vi "nivision_savepng.vi"(6 "Use bit depth? (false)":bool, 7 "Color Palette":cluster{"Red":u8, "Green":u8, "Blue":u8}[](array[cluster]), 8 "error in (no error)":errorcluster, 9 "Image Quality":u32=750 max=1000 step=10, 10 "File Path":path, 11 "Image":T1) -> (0 "error out":errorcluster, 3 "Image Out (duplicate)":T1)   [LabVIEW 2019]
uses:
  <vilib>/vision/Image Controls.llb/IMAQ Image.ctl
  nivision.dll
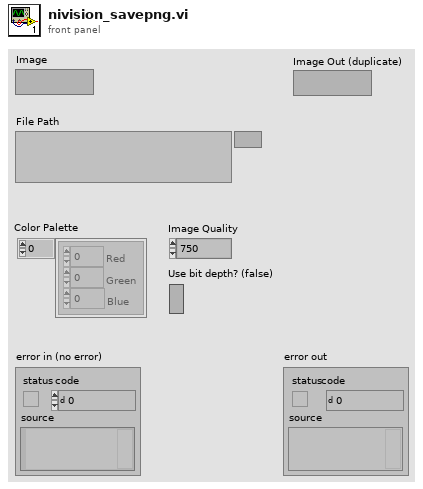
[diagram p1: front panel]
types:
  T1 = typedef "IMAQ Image.ctl" = refnum<image>
  T2 = cluster{"Image Quality":u32, "Use bit depth? (false)":bool}
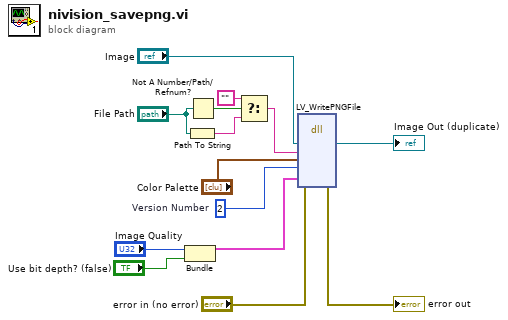
[diagram p0: block diagram]
diagram:
  w12 = 2  # Version Number
  n1 = Bundle("Image Quality"="Image Quality", "Use bit depth? (false)"="Use bit depth? (false)") -> (w8:T2)  [unwired: 1 out]
  n2 = Path To String(path="File Path") -> (string=w4:string)
  n3 = Not A Number/Path/Refnum?(number/path/refnum="File Path") -> (NaN/Path/Refnum?=w3:bool)
  n4 = Select(t="", s=w3, f=w4) -> (s? t:f=w2:string)
  n5 = dll-call lib="NIVision.dll" fn="LV_WritePNGFile"("SourceImage"="Image", "FilePath"=w2, "ColorPalette"="Color Palette", "Version"=w12, "options"=w8, "Error"="error in (no error)") -> ("SourceImage"=→"Image Out (duplicate)":T1, "Error"=→"error out":errorcluster)  [unwired: 6 in, 4 out]
